vi "Execice1.vi"() -> ()   [LabVIEW 2018]
panel:
  out "X/Y":dbl format="%#.3g"
  out "X*Y":dbl format="%#.3g"
  out "X-Y":dbl format="%#.3g"
  out "X+Y":dbl format="%#.3g"
  in  "Numeric":dbl min=0.0 max=9.0
  in  "Slide":dbl(slide) min=0.0 max=9.0 scale=0.0..9.0
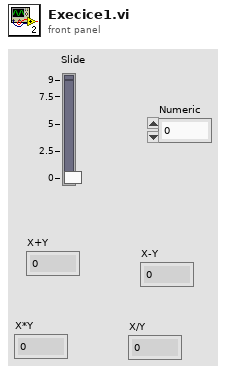
[diagram p1: front panel]
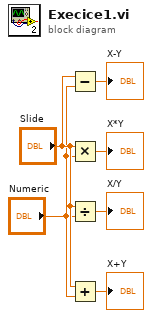
[diagram p0: block diagram]
diagram:
  n1 = Subtract(x="Slide", y="Numeric") -> (x-y=→"X-Y":dbl)
  n2 = Multiply(x="Slide", y="Numeric") -> (x*y=→"X*Y":dbl)
  n3 = Divide(x="Slide", y="Numeric") -> (x/y=→"X/Y":dbl)
  n4 = Add(x="Slide", y="Numeric") -> (x+y=→"X+Y":dbl)
